vi "Compute.vi"(7 "SHA-1":refnum<class "SHA-1.lvclass">, 10 "data":u8[](array[numeric]) format="%02x") -> (2 "hash":u8[](array[numeric]) format="%02x")   [LabVIEW 2013, in "SHA-1.lvlib" / "SHA-1.lvclass"]
doc: "This VI contains the core of the MD5 algorithm."
uses:
  SHA-1.lvclass
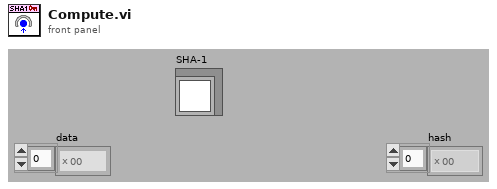
[diagram p1: front panel]
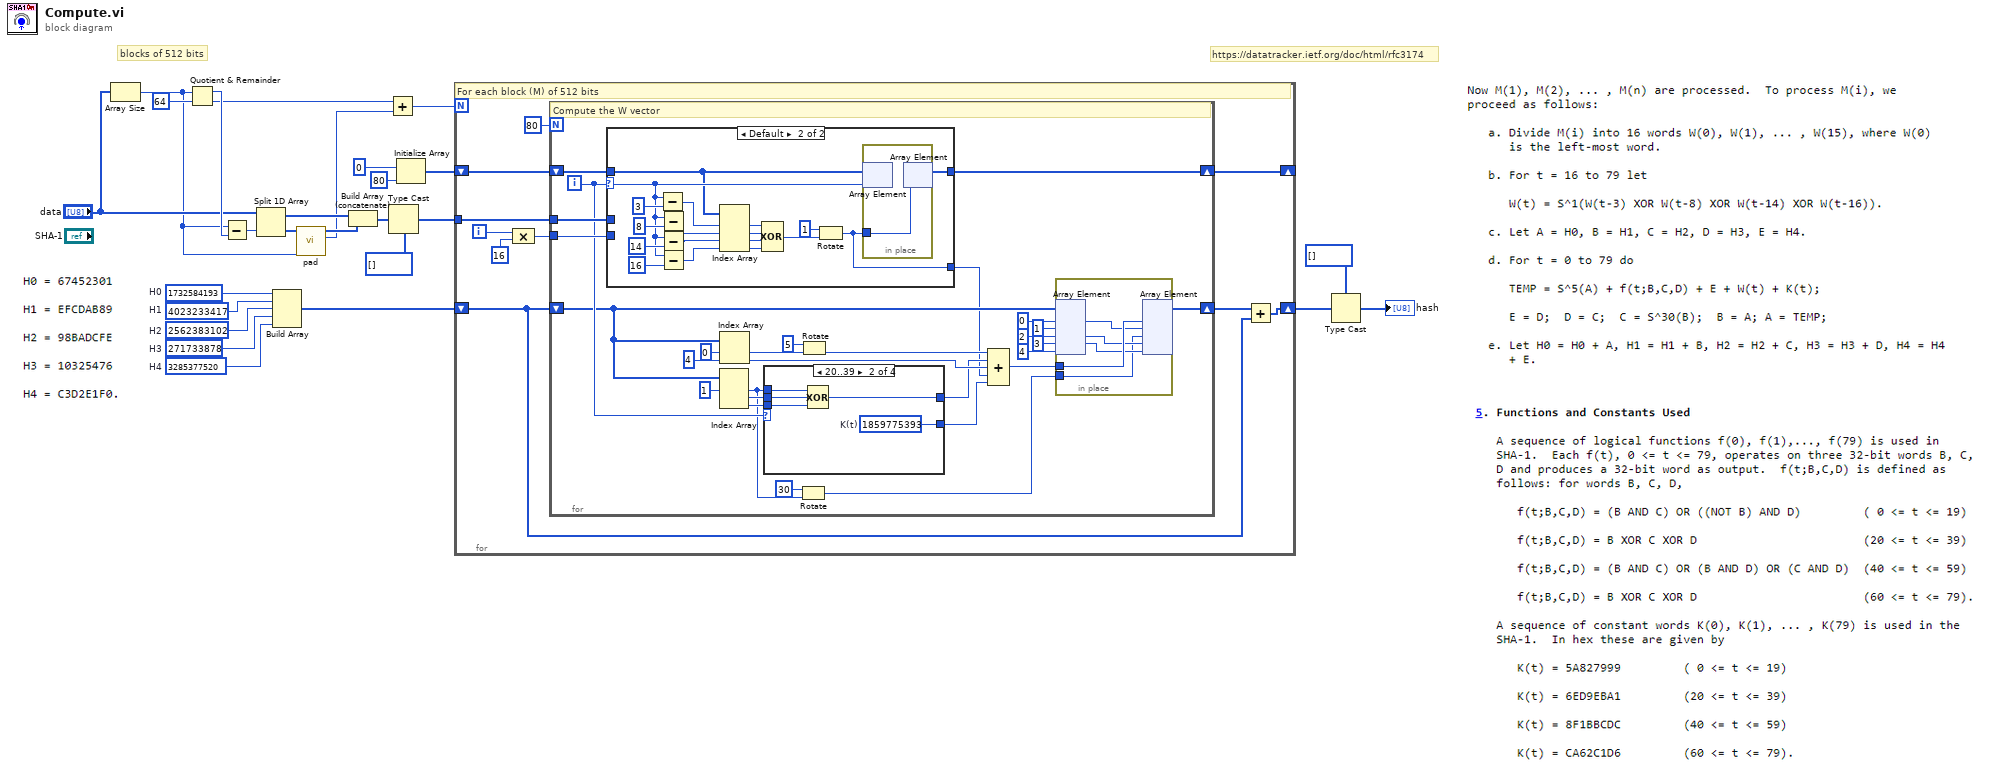
[diagram p0: block diagram]
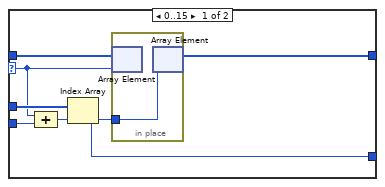
[diagram p2: hidden frame]
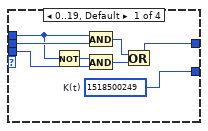
[diagram p3: hidden frame]
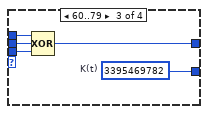
[diagram p4: hidden frame]
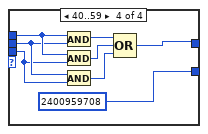
[diagram p5: hidden frame]
diagram:
  w10 = u32 3285377520  # H4
  w11 = u32 271733878  # H3
  w12 = u32 2562383102  # H2
  w13 = u32 4023233417  # H1
  w14 = u32 1732584193  # H0
  # "blocks of 512 bits"
  # "https://datatracker.ietf.org/doc/html/rfc3174"
  n1 = Array Size(array="data") -> (size(s)=w7:i32)
  n2 = Quotient & Remainder(x=w7, y=64) -> (x-y*floor(x/y)=w26:i32, floor(x/y)=w4:i32)
  n3 = Subtract(x=w7, y=w26) -> (x-y=w20:i32)
  n4 = Split 1D Array(array="data", index=w20) -> (first subarray=w18:u8[], second subarray=w6:u8[])
  n5 = Build Array(w14, w13, w12, w11, w10) -> (w1:u32[])
  n6 = call "pad.vi"("data length"=w7, "Last Block"=w6) -> ("blocks"=w3:i32, "Padding"=w5:u8[])  [unwired: 8 in]
  n7 = Build Array (concatenate)(w18, w5) -> (w17:u8[])
  n8 = Add(x=w4, y=w3) -> (x+y=w2:i32)
  n9 = Type Cast(type=u32[] [] ("U32"), x=w17) -> (*(type *) &x=w16:u32[])
  n10 = Initialize Array(u32 0, 80) -> (w22:u32[])
  n11 = for {
    N: w2 -> [_]
    tunnel: w16 -> [w33]
    shift-right: [w34] -> _
    shift-left: w22 -> [w29]
    shift-right: [w30] -> w9
    shift-left: w1 -> [w31]
    i -> [w36]
    # "For each block (M) of 512 bits"
    n12 = Compound Arithmetic op=MULTIPLY(w36, 16) -> (w27:i32)
    n13 = for {
      N: 80 -> [_]
      shift-right: [w61] -> w34
      shift-left: w29 -> [w62]
      tunnel: w33 -> [w64]
      tunnel: w27 -> [w63]
      shift-right: [w41] -> w32
      shift-left: w31 -> [w50]
      i -> [w60]
      # "Compute the W vector"
      n14 = case shown="Default" w60 {
        selector: w60 -> [w71 w90]
        tunnel: w64 -> [w76 _]
        tunnel: w63 -> [w75 _]
        tunnel: w62 -> [w74 w85]
        tunnel: [w73 w95] -> w61
        tunnel: [w72 w78] -> w37
        frame 0..15 {
          n15 = Compound Arithmetic op=ADD(w71, w75) -> (w70:i32)
          n16 = Index Array(array=w76, index=w70) -> (element=w72:u32)
          n17 = in-place {
            in-place-border: w72 -> [w77]
            n18 = in-place-array #1(w74, w71) -> ()  [unwired: 1 out]
            n19 = in-place-array #1(w77) -> (w73:u32[])  [unwired: 1 out]
          }
        }
        frame Default {
          n20 = Subtract(x=w90, y=3) -> (x-y=w84:i32)
          n21 = Subtract(x=w90, y=8) -> (x-y=w83:i32)
          n22 = Subtract(x=w90, y=14) -> (x-y=w82:i32)
          n23 = Subtract(x=w90, y=16) -> (x-y=w81:i32)
          n24 = Index Array(array=w85, index #1=w84, index #2=w83, index #3=w82, index #4=w81) -> (element #1=w89:u32, element #2=w88:u32, element #3=w87:u32, element #4=w86:u32)
          n25 = Compound Arithmetic op=XOR(w89, w88, w87, w86) -> (w79:u32)
          n26 = Rotate(1:w79, 2:i8 1 ("y")) -> (0:w78:u32)
          n27 = in-place {
            in-place-border: w78 -> [w96]
            n28 = in-place-array #2(w85, w90) -> ()  [unwired: 1 out]
            n29 = in-place-array #2(w96) -> (w95:u32[])  [unwired: 1 out]
          }
        }
      }
      n30 = Index Array(array=w50, index #1=1 ("index")) -> (element #1=w48:u32, element #2=w53:u32, element #3=w52:u32)  [unwired: 2 in]
      n31 = Index Array(array=w50, index #1=0 ("index"), index #2=4 ("index")) -> (element #1=w56:u32, element #2=w39:u32)
      n32 = case shown="20..39" w60 {
        tunnel: w48 -> [w99 w109 w114 w122]
        tunnel: w53 -> [w100 w108 w113 w121]
        tunnel: w52 -> [w101 w107 w112 w120]
        tunnel: [w98 w105 w110 w116] -> w38
        tunnel: [w97 w106 w111 u32 2400959708] -> w40
        frame 0..19, Default {
          w97 = u32 1518500249  # K(t)
          n33 = Not(x=w99) -> (.not. x?=w104:u32)
          n34 = And(x=w99, y=w100) -> (x .and. y?=w102:u32)
          n35 = And(x=w104, y=w101) -> (x .and. y?=w103:u32)
          n36 = Or(x=w102, y=w103) -> (x .or. y?=w98:u32)
        }
        frame 20..39 {
          w106 = u32 1859775393  # K(t)
          n37 = Compound Arithmetic op=XOR(w109, w108, w107) -> (w105:u32)
        }
        frame 60..79 {
          w111 = u32 3395469782  # K(t)
          n38 = Compound Arithmetic op=XOR(w114, w113, w112) -> (w110:u32)
        }
        frame 40..59 {
          n39 = And(x=w122, y=w121) -> (x .and. y?=w119:u32)
          n40 = And(x=w122, y=w120) -> (x .and. y?=w118:u32)
          n41 = And(x=w121, y=w120) -> (x .and. y?=w117:u32)
          n42 = Compound Arithmetic op=OR(w119, w118, w117) -> (w116:u32)
        }
      }
      n43 = Rotate(1:w48, 2:i8 30 ("y")) -> (0:w42:u32)
      n44 = Rotate(1:w56, 2:i8 5 ("y")) -> (0:w55:u32)
      n45 = Compound Arithmetic op=ADD(w55, w38, w39, w37, w40) -> (w51:u32)
      n46 = in-place {
        in-place-border: w51 -> [w69]
        in-place-border: w42 -> [w65]
        n47 = in-place-array #3(w50, 0, 1, 2, 3, 4) -> (w68:u32, w67:u32, w66:u32)  [unwired: 2 out]
        n48 = in-place-array #3(w69, w68, w65, w67, w66) -> (w41:u32[])  [unwired: 5 out]
      }
    }
    n49 = Add(x=w32, y=w31) -> (x+y=w30:u32[])
  }
  n50 = Type Cast(type=u8[] [], x=w9) -> (*(type *) &x=→"hash":u8[])
